vi "test - remove keys in sperated but same name session.vi"(8 "error in (no error)":errorcluster, 11 "TestCase in":refnum<class "labview-config-library.lvclass">) -> (0 "error out":errorcluster, 3 "TestCase out":refnum<class "labview-config-library.lvclass">)   [LabVIEW 2017, in "labview-config-library.lvclass"]
uses:
  labview-config-library.lvclass
  <vilib>/addons/_JKI Toolkits/VI Tester/TestCase.llb/TestCase.lvclass
  INI-Static-Variable-Support/LabVIEW-Config/LabVIEW-Config.lvclass
  <userlib>/_NEVSTOP/Communicable State Machine(CSM)/Communicable State Machine.lvlib
  C:/Program Files (x86)/National Instruments/LabVIEW 2017/vi.lib/addons/_JKI Toolkits/VI Tester/TestCase.llb/TestCase.lvclass
panel:
  in  "Tab Control":enum32{"Page 1", "Page 2", "Page 3"}(tab)
  out "Section Names":string[](array[string])
  out "Key Names":string[](array[string])
  out "Key Names 2":string[](array[string])
  out "text":string
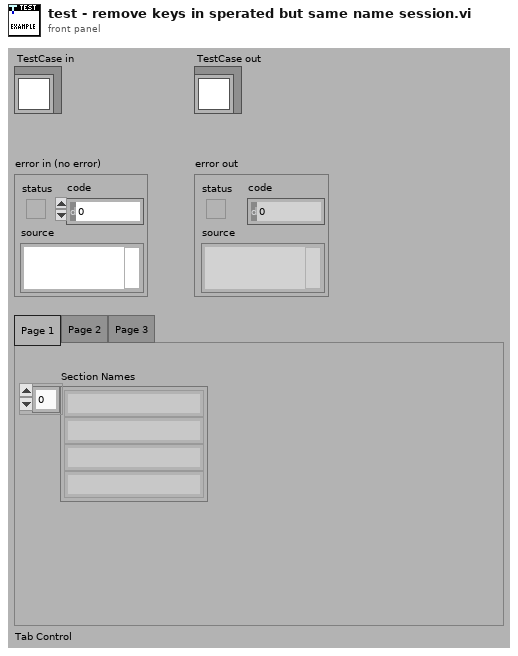
[diagram p1: front panel]
types:
  T1 = typedef "LabVIEW-Config.lvlib/LabVIEW-Config.lvclass/Config.ctl" = cluster{"Path":path, "Lines":string[], "Tokens":T2[], "Modified?":bool, "Cache":cluster{"Valid?":bool, "Key Information":T3[]}}
  T2 = typedef "LabVIEW-Config.lvlib/LabVIEW-Config.lvclass/LineToken.ctl" = enum8{"comment", "section", "key", "more"}
  T3 = typedef "LabVIEW-Config.lvlib/LabVIEW-Config.lvclass/KeyInfo.ctl" = cluster{"Key Indexes":cluster{"Indexes":i32[]}[], "Session Found?":bool, "Key found?":bool, "Session Index":i32}
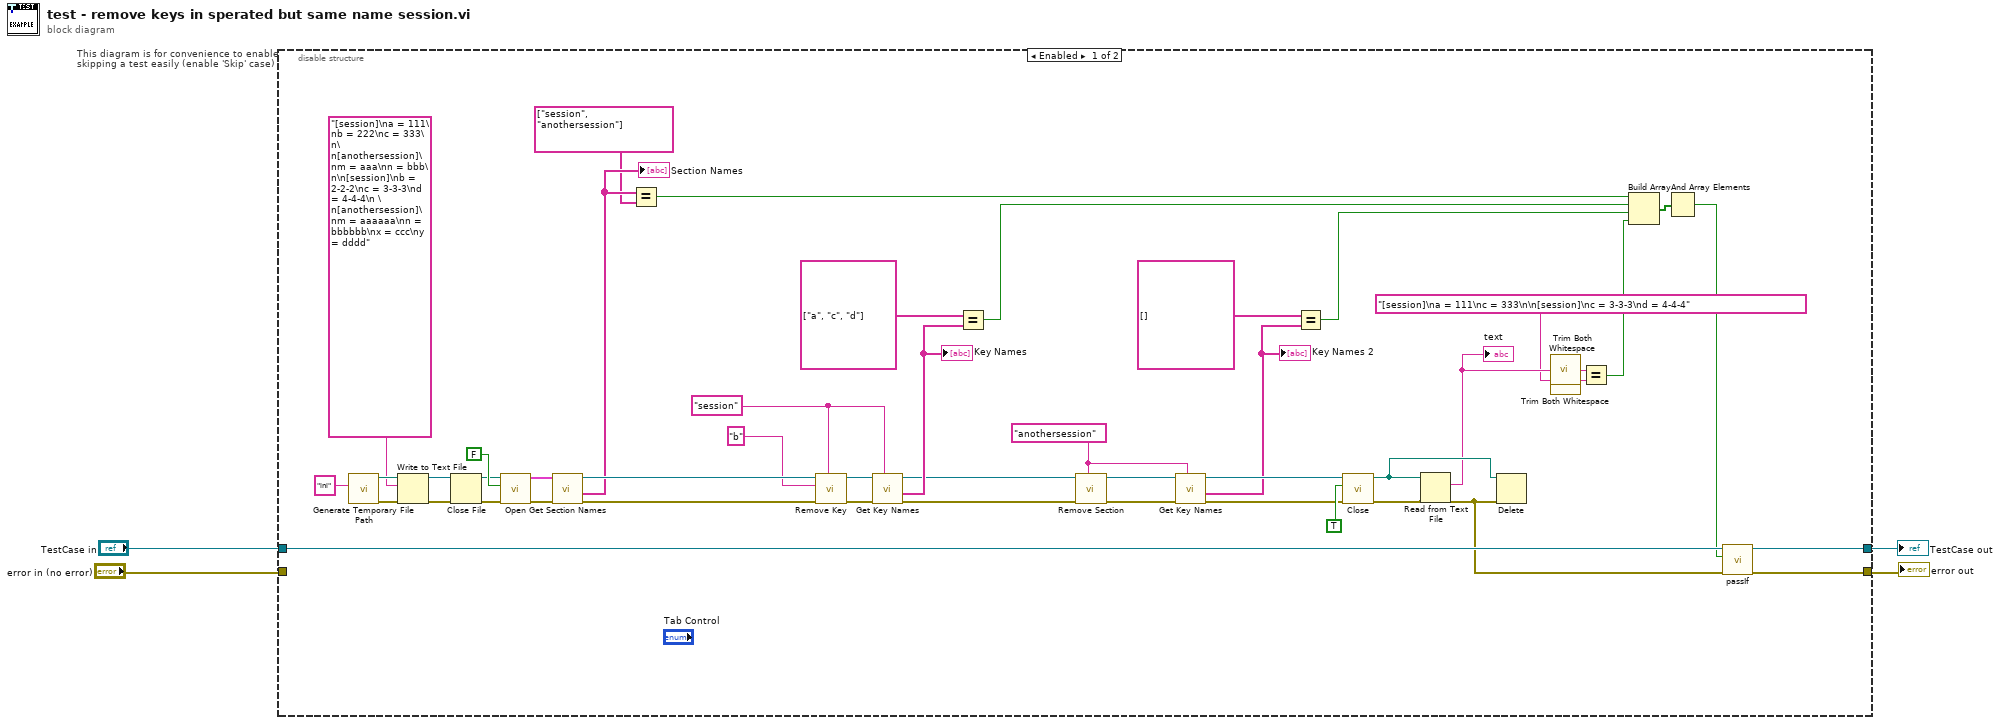
[diagram p0: block diagram]
diagram:
  n1 = disable-structure "This diagram is for convenience to enable skipping a test easily (enable 'Skip' case)" shown="Enabled" {
    disable-tunnel: "TestCase in" -> [w51 w55]
    disable-tunnel: [w50 w53] -> w1
    disable-tunnel: [w49 w54] -> w3
    disable-tunnel: "error in (no error)" -> [_ w52]
    frame Enabled {
      w18 = "anothersession"
      w26 = "session" ("Section Name")
      # "Create temporary ini file"
      n2 = call <vilib>:"Generate Temporary File Path.vi"("Temporary File Extension (tmp)"="ini") -> ("error out"=w46:errorcluster, "Unique Temporary File Path"=w43:path)  [unwired: 9 in]
      n3 = Write to Text File(file (use dialog)=w43, text="[session]\na = 111\nb = 222\nc = 333\n\n[anothersession]\nm = aaa\nn = bbb\n\n[session]\nb = 2-2-2\nc = 3-3-3\nd = 4-4-4\n \n[anothersession]\nm = aaaaaa\nn = bbbbbb\nx = ccc\ny = dddd", error in=w46) -> (refnum out=w42:refnum<file>, error out=w44:errorcluster)  [unwired: 1 in, 1 out]
      n4 = Close File(refnum=w42, error in=w44) -> (path=w39:path, error out=w40:errorcluster)
      n5 = call "Open.vi"("error in (no error)"=w40, "Create if not exists? (T)"=FALSE, "Path"=w39) -> ("error out"=w37:errorcluster, "Config"=w38:T1)  [unwired: 5 in, 2 out]
      n6 = call "Get Section Names.vi"("error in (no error)"=w37, "Config in"=w38) -> ("error out"=w35:errorcluster, "Section Names"=w34:string[], "Config out"=w36:refnum<class "LabVIEW-Config.lvclass">)  [unwired: 7 in]
      "Section Names" <- w34
      n7 = Equal?(x=w34, y=string[] ["session", "anothersession"]) -> (x = y?=w32:bool)
      n8 = call "Remove Key.vi"("Section Name"=w26, "error in (no error)"=w35, "Key Name"="b", "Config in"=w36) -> ("error out"=w27:errorcluster, "Config out"=w28:refnum<class "LabVIEW-Config.lvclass">)  [unwired: 5 in, 1 out]
      n9 = call "Get Key Names.vi"("Section Name"=w26, "error in (no error)"=w27, "Config in"=w28) -> ("error out"=w21:errorcluster, "Key Names"=w24:string[], "Config out"=w22:refnum<class "LabVIEW-Config.lvclass">)  [unwired: 5 in, 1 out]
      "Key Names" <- w24
      n10 = Equal?(x=string[] ["a", "c", "d"] ("Key Names"), y=w24) -> (x = y?=w23:bool)
      n11 = call "Remove Section.vi"("Section Name"=w18, "error in (no error)"=w21, "Config in"=w22) -> ("error out"=w19:errorcluster, "Config out"=w20:refnum<class "LabVIEW-Config.lvclass">)  [unwired: 6 in, 1 out]
      n12 = call "Get Key Names.vi"("Section Name"=w18, "error in (no error)"=w19, "Config in"=w20) -> ("error out"=w17:errorcluster, "Key Names"=w14:string[], "Config out"=w16:refnum<class "LabVIEW-Config.lvclass">)  [unwired: 5 in, 1 out]
      "Key Names 2" <- w14
      n13 = Equal?(x=string[] [] ("Key Names"), y=w14) -> (x = y?=w13:bool)
      n14 = call "Close.vi"("error in (no error)"=w17, "Write if modified? (T)"=TRUE, "Config"=w16) -> ("error out"=w11:errorcluster, "Path"=w12:path)  [unwired: 7 in]
      n15 = Read from Text File(file (use dialog)=w12, error in=w11) -> (text=w9:string, error out=w10:errorcluster)  [unwired: 2 in, 2 out]
      "text" <- w9
      n16 = Delete(path (use dialog)=w12, error in=w10) -> ()  [unwired: 3 in, 3 out]
      n17 = call <userlib>:"Trim Both Whitespace.vi"("string"=w9) -> ("trimmed string"=w6:string)  [unwired: 1 in]
      n18 = call <userlib>:"Trim Both Whitespace.vi"("string"="[session]\na = 111\nc = 333\n\n[session]\nc = 3-3-3\nd = 4-4-4" ("y")) -> ("trimmed string"=w5:string)  [unwired: 1 in]
      n19 = Equal?(x=w6, y=w5) -> (x = y?=w7:bool)
      n20 = Build Array(w32, w23, w13, w7) -> (w31:bool[])
      n21 = And Array Elements(Boolean array=w31) -> (logical AND=w30:bool)
      n22 = call-dynamic "passIf.vi"("error in (no error)"=w10, "pass"=w30, "TestCase in"=w51) -> ("error out"=w49:errorcluster, "TestCase out"=w50:refnum<class "labview-config-library.lvclass">)  [unwired: 7 in]
    }
    frame Disabled {
      # "skip test result while test is under development"
      n23 = call <vilib>:"skip.vi"("error in (no error)"=w52, "TestCase in"=w55) -> ("error out"=w54:errorcluster, "TestCase out"=w53:refnum<class "labview-config-library.lvclass">)  [unwired: 8 in]
    }
  }
  "error out" <- w3
  "TestCase out" <- w1
